vi "FRU PROGRAMMING TOOLKIT - Copy.vi"() -> ()   [LabVIEW 2016]
doc: "This EEPROM example shows a more generalized way to use the I2C basic API to write data. It allows the user to change the following parameters: page size, write delay, the endianness of the address bytes, and the number of bytes in an address.\n\nThe parameters will have the following effects:\n\nTarget Page Size (bytes): This places an additional constraint on the amount of bytes written. The smaller value will be used, and that number of bytes written.\nWrite Delay Between Pages (ms): This will force a mandatory delay after writing bytes to a device.\nData Address Width: This will allow the user to specify the EEPROM Data Address as either 1 or 2 bytes.\nData Address Endianness: This control will change the ordering of the bytes in the EEPROM Data Address, note that this only has an effect if there are 2 bytes in the address.\n\nSince the I2C SDA and SCL lines are open-drain, they must be pulled up to the required reference voltage of your slave by connecting an appropriate resistor (2k-5k) between SCL and your reference voltage and SDA and your reference voltage. For NI-845x Hardware that contain internal pull-ups, you can use these. Otherwise, you need to use external pullups.\n\nFor connection information see the NI-845x Hardware and Software manual and the manual for your specific EEPROM."
uses:
  Type Definitions/I2C Slave Configuration.ctl
  Type Definitions/I2C Device Configuration.ctl
  <vilib>/ni845x/ni845x.llb/ni845xControl.ctl
  Type Definitions/FRU Type.ctl
  Type Definitions/FRU Information.ctl
  Type Definitions/Unique FRU Input.ctl
  Type Definitions/I2C Data Cluster.ctl
  <vilib>/Utility/miscctls.llb/LVRectTypeDef.ctl
  <vilib>/ni845x/ni845x.llb/ni845xI2cConfiguration.ctl
  Type Definitions/I2C Data Address Cluster.ctl
  <vilib>/ni845x/ni845x.llb/NI-845x Close Device Reference.vi
panel:
  out "Front Panel Window:Panel Bounds":T1
  in  "Test Type":enum32{"Standard", "Advanced"}(tab)
  in  "FRU Type":T2
  in  "Unique FRU Input":T3
  in  "I2C Data Cluster":T4={"Address Byte"=0, "Number of Bytes"=0, "Page Size in Bytes"=128, "Data Byte"=[], "Write Delay Between Pages (ms)"=4} {"Data Byte" format="%02x"; "Address Byte" format="%04x"}
  out "PASS":bool
  out "FRU Out":T5
  out "Read Byte":u8[](array[numeric]) format="%02x"
  in  "READ":bool
  in  "Device in":T6="USB0::0x3923::0x7166::01EEC019::RAW"
  out "error out":errorcluster
  in  "INIT":bool
  out "TESTING":bool
  in  "error in (no error)":errorcluster
  in  "EXIT":bool
  in  "CONNECT":bool
  in  "START TEST":bool
  in  "DISCONNECT":bool
  out "Written Byte":u8[](array[numeric]) format="%02x"
  out "Device Out":T6
  in  "I2C Device Configuration":T7={"I²C Pullup Enable"=FALSE, "Timeout Value (ms)"=50000}
  in  "WRITE":bool
  in  "I2C Slave Configuration":T8={"Address"=80, "Clock Rate (kHz)"=100, "Address Size"=0} {"Address Size" items=["7 Bits", "10 Bits"]; "Address" format="%.0x"}
  # "FRU Programming Toolkit"
  # "SOLAHD SCM"
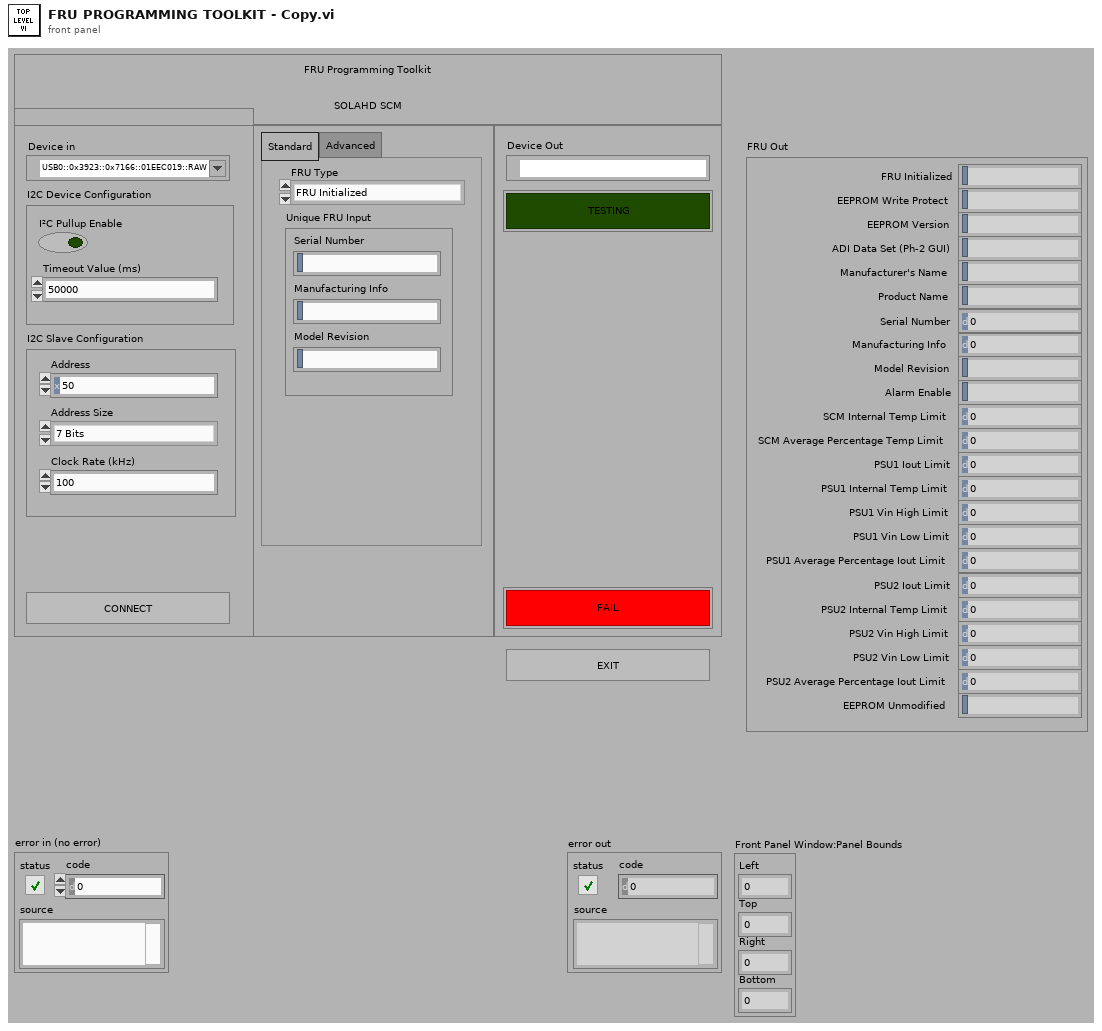
[diagram p1: front panel]
types:
  T1 = typedef "LVRectTypeDef.ctl" = cluster{"Left":i16, "Top":i16, "Right":i16, "Bottom":i16}
  T2 = typedef "FRU Type.ctl" = enum16{"FRU Initialized", "EEROM Write Protect", "EEPROM Version", "ADI Data Set (Ph-2 GUI)", "Manufacturer's Name", "Product Name", "Serial Number", "Manufacturing Info", "Model Revision", "Alarm Enable", "SCM Internal Temp Limit", "SCM Average Percentage Temp Limit", "PSU1 Iout Limit", "PSU1 Internal Temp Limit", "PSU1 Vin High Limit", "PSU1 Vin Low Limit", "PSU1 Average Percentage Iout Limit", "PSU2 Iout Limit", "PSU2 Internal Temp Limit", "PSU2 Vin High Limit", "PSU2 Vin Low Limit", "PSU2 Average Percentage Iout Limit", "EEPROM Unmodified"}
  T3 = typedef "Unique FRU Input.ctl" = cluster{"Serial Number":string, "Manufacturing Info":string, "Model Revision":string}
  T4 = typedef "I2C Data Cluster.ctl" = cluster{"Address Byte":u16, "Number of Bytes":u32, "Page Size in Bytes":u32, "Data Byte":u8[], "Write Delay Between Pages (ms)":u32}
  T5 = typedef "FRU Information.ctl" = cluster{"FRU Initialized":string, "EEPROM Write Protect":string, "EEPROM Version":string, "ADI Data Set (Ph-2 GUI)":string, "Manufacturer's Name":string, "Product Name":string, "Serial Number":u32, "Manufacturing Info":u32, "Model Revision":string, "Alarm Enable":string, "SCM Internal Temp Limit":u32, "SCM Average Percentage Temp Limit":u32, "PSU1 Iout Limit":u32, "PSU1 Internal Temp Limit":u32, "PSU1 Vin High Limit":u32, "PSU1 Vin Low Limit":u32, "PSU1 Average Percentage Iout Limit":u32, "PSU2 Iout Limit":u32, "PSU2 Internal Temp Limit":u32, "PSU2 Vin High Limit":u32, "PSU2 Vin Low Limit":u32, "PSU2 Average Percentage Iout Limit":u32, "EEPROM Unmodified":string}
  T6 = typedef "ni845xControl.ctl" = refnum<k21>
  T7 = typedef "I2C Device Configuration.ctl" = cluster{"I²C Pullup Enable":bool, "Timeout Value (ms)":u32}
  T8 = typedef "I2C Slave Configuration.ctl" = cluster{"Address":u16, "Clock Rate (kHz)":u16, "Address Size":i32}
  T9 = typedef "ni845xI2cConfiguration.ctl" = refnum<k20>
  T10 = typedef "I2C Data Address Cluster.ctl" = cluster{"Data Address Endianness":bool, " Data Address Width":enum16{"1 Byte", "2 Byte"}}
  T11 = enum16{"Always On", "Always Off", "Off While Running"}
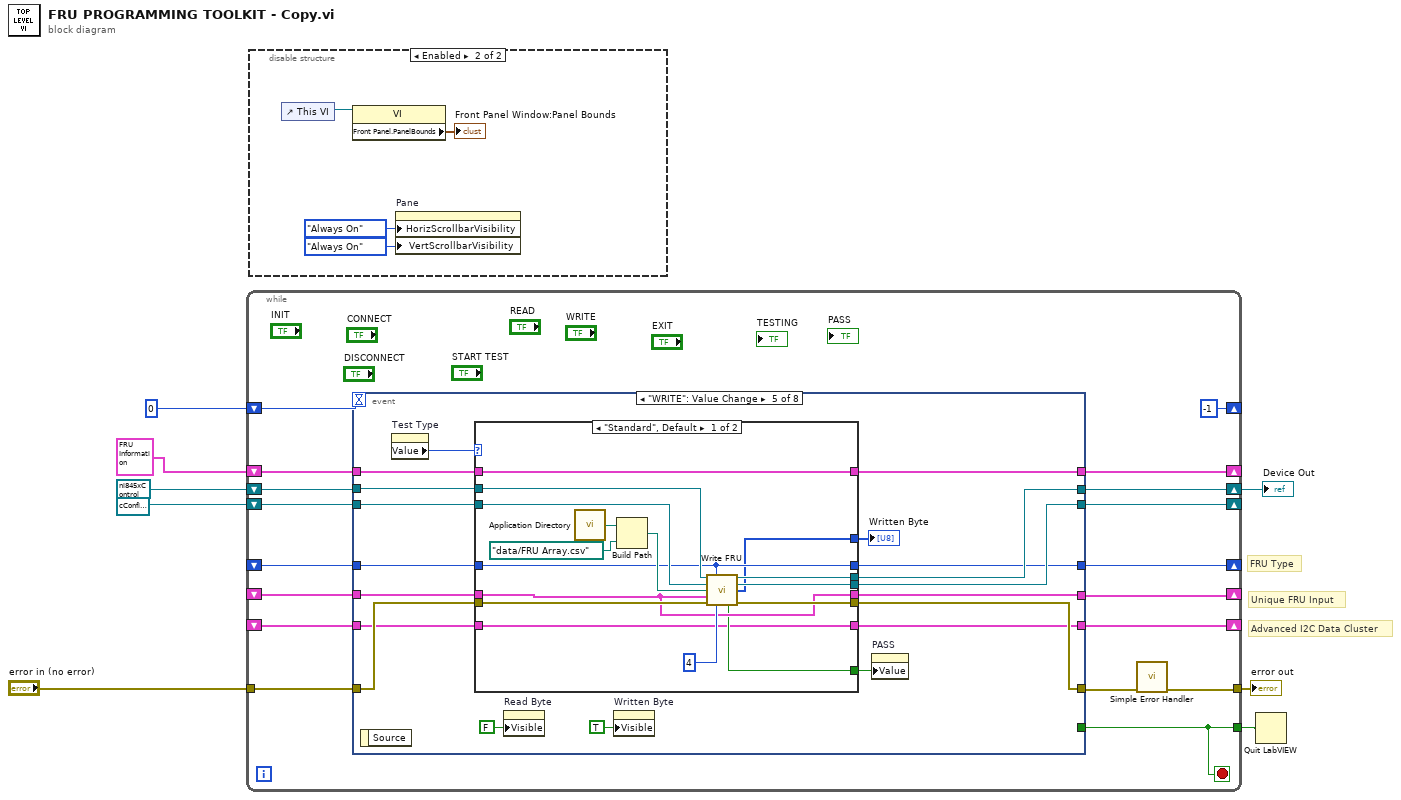
[diagram p0: block diagram]
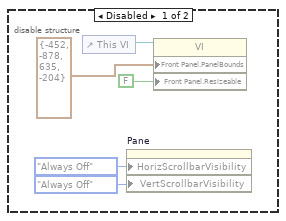
[diagram p2: hidden frame]
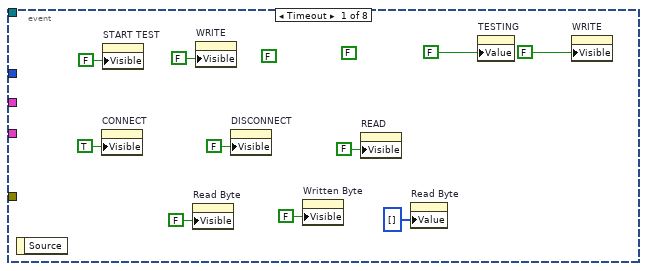
[diagram p3: hidden frame]
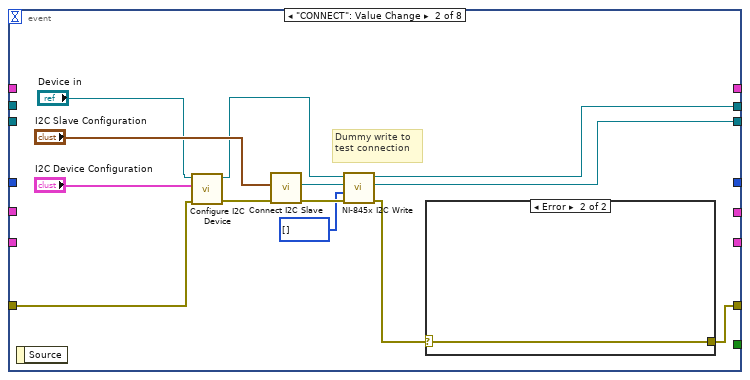
[diagram p4: hidden frame]
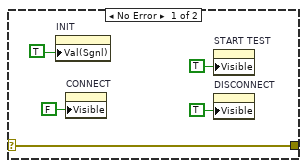
[diagram p5: hidden frame]
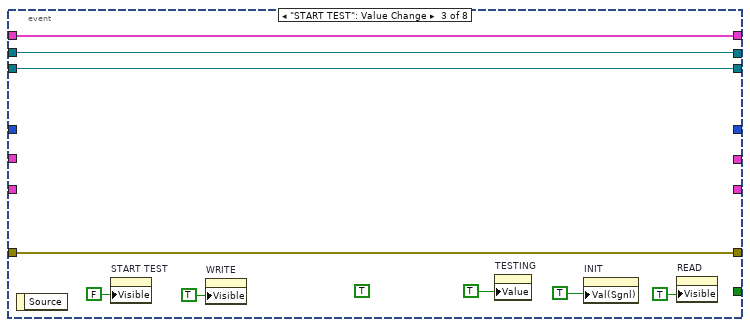
[diagram p6: hidden frame]
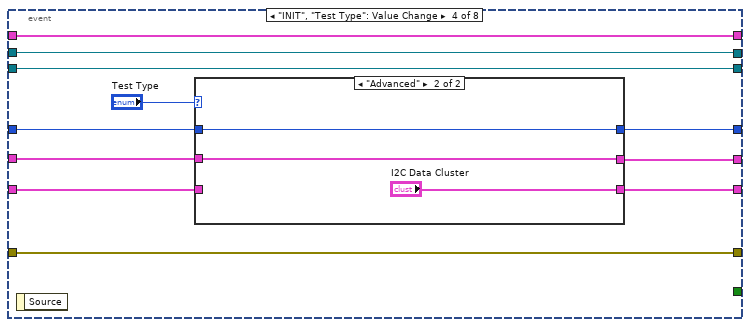
[diagram p7: hidden frame]
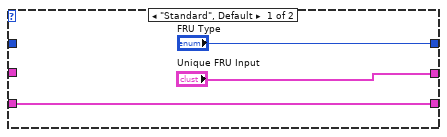
[diagram p8: hidden frame]
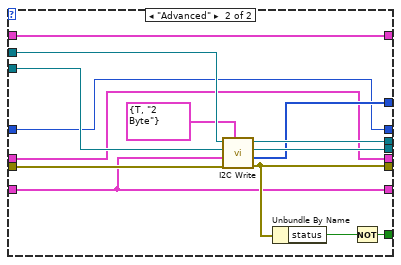
[diagram p9: hidden frame]
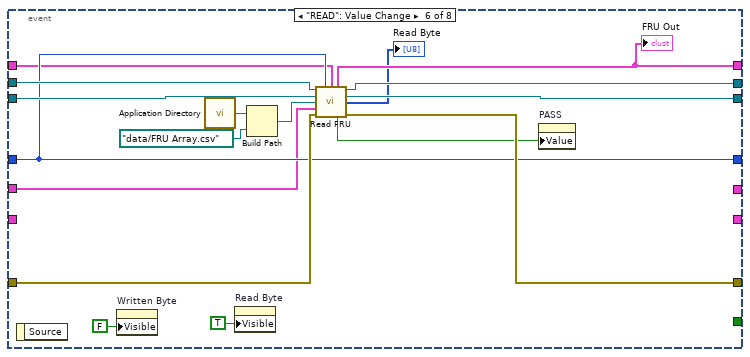
[diagram p10: hidden frame]
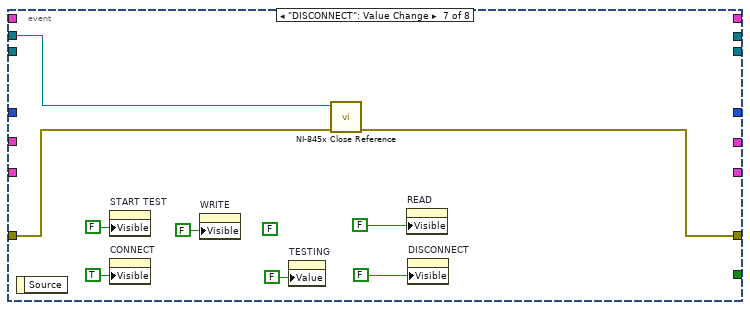
[diagram p11: hidden frame]
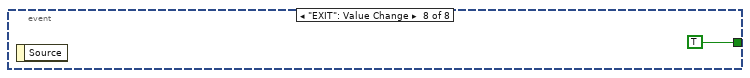
[diagram p12: hidden frame]
diagram:
  # "Advanced I2C Data Cluster"
  # "Unique FRU Input"
  # "FRU Type"
  n1 = while {
    tunnel: [w26] -> w8
    shift-right: [w23] -> _
    shift-left: T9 refnum ("i2c configuration") -> [w20]
    shift-right: [w25] -> w7
    shift-left: T6 refnum ("Device out") -> [w17]
    shift-right: [-1] -> _
    shift-left: 0 -> [w19]
    tunnel: "error in (no error)" -> [w24]
    tunnel: [w21] -> w3
    shift-right: [w16] -> _
    shift-left: T5 {"FRU Initialized"="", "EEPROM Write Protect"="", "EEPROM Version"="", "ADI Data Set (Ph-2 GUI)"="", "Manufacturer's Name"="", "Product Name"="", "Serial Number"=0, "Manufacturing Info"=0, "Model Revision"="", "Alarm Enable"="", "SCM Internal Temp Limit"=0, "SCM Average Percentage Temp Limit"=0, "PSU1 Iout Limit"=0, "PSU1 Internal Temp Limit"=0, "PSU1 Vin High Limit"=0, "PSU1 Vin Low Limit"=0, "PSU1 Average Percentage Iout Limit"=0, "PSU2 Iout Limit"=0, "PSU2 Internal Temp Limit"=0, "PSU2 Vin High Limit"=0, "PSU2 Vin Low Limit"=0, "PSU2 Average Percentage Iout Limit"=0, "EEPROM Unmodified"=""} ("FRU Information Out") -> [w15]
    shift-right: [w14] -> _
    shift-left: _ -> [w13]
    shift-right: [w12] -> _
    shift-left: _ -> [w11]
    shift-right: [w10] -> _
    shift-left: _ -> [w9]
    stop <- w26 stop-if-true
    n2 = event shown="[4] \"WRITE\": Value Change" {
      selector: _ -> [_ _ _ _ _ _ _ _]
      dyn-events: _ -> [_ _ _ _ _ _ _ _]
      timeout: w19 -> [_ _ _ _ _ _ _ _]
      tunnel: [_ _ _ _ _ _ _ TRUE] -> w26
      tunnel: [_ w43 w59 w74 w94 w145 _ _] -> w25
      tunnel: w17 -> [_ _ w59 w74 w96 w147 w149 _]
      tunnel: [_ w39 w64 w75 w97 w141 w152 _] -> w22
      tunnel: w24 -> [_ w46 w64 w75 w100 w144 w148 _]
      tunnel: [_ w42 w56 w71 w93 w137 _ _] -> w23
      tunnel: w20 -> [_ _ w56 w71 w95 w146 _ _]
      tunnel: [_ _ w57 w72 w89 w133 _ _] -> w16
      tunnel: w15 -> [_ _ w57 w72 w90 w135 _ _]
      tunnel: [_ _ _ w73 w88 w136 _ _] -> w14
      tunnel: w13 -> [_ _ _ w66 w92 w136 _ _]
      tunnel: [_ _ _ w70 w86 _ _ _] -> w12
      tunnel: w11 -> [_ _ _ w67 w91 w132 _ _]
      tunnel: [_ _ _ w68 w83 _ _ _] -> w10
      tunnel: w9 -> [_ _ _ w65 w87 _ _ _]
      event Timeout {
        (unwired) FALSE ("Visible")
        (unwired) FALSE ("Visible")
        n3 = event-data() -> ()  [unwired: 1 in, 1 out]
        n4 = property on="CONNECT" class="Bool"("Visible"=TRUE) -> ()  [unwired: 2 in, 2 out]
        n5 = property on="START TEST" class="Bool"("Visible"=FALSE) -> ()  [unwired: 2 in, 2 out]
        n6 = property on="Read Byte" class="Arr (strict)"("Visible"=FALSE) -> ()  [unwired: 2 in, 2 out]
        n7 = property on="WRITE" class="Bool"("Visible"=FALSE) -> ()  [unwired: 2 in, 2 out]
        n8 = property on="DISCONNECT" class="Bool"("Visible"=FALSE) -> ()  [unwired: 2 in, 2 out]
        n9 = property on="Written Byte" class="Arr (strict)"("Visible"=FALSE) -> ()  [unwired: 2 in, 2 out]
        n10 = property on="READ" class="Bool"("Visible"=FALSE) -> ()  [unwired: 2 in, 2 out]
        n11 = property on="Read Byte" class="Arr (strict)"("Value"=u8[] []) -> ()  [unwired: 2 in, 2 out]
        n12 = property on="TESTING" class="Bool (strict)"("Value"=FALSE ("TESTING")) -> ()  [unwired: 2 in, 2 out]
        n13 = property on="WRITE" class="Bool"("Visible"=FALSE) -> ()  [unwired: 2 in, 2 out]
      }
      event "CONNECT": Value Change {
        # "Dummy write to test connection"
        n14 = event-data() -> ()  [unwired: 1 in, 1 out]
        n15 = call "Configure I2C Device.vi"("error in (no error)"=w46, "I2C Device Configuration"="I2C Device Configuration", "Device In"="Device in") -> ("error out"=w47:errorcluster, "Device out"=w41:T6)  [unwired: 7 in]
        n16 = call "Connect I2C Slave.vi"("error in (no error)"=w47, "I2C Slave Configuration"="I2C Slave Configuration") -> ("error out"=w45:errorcluster, "i2c configuration"=w44:T9)  [unwired: 8 in]
        n17 = call <vilib>:"NI-845x I2C Write.vi"("error in (no error)"=w45, "write data"=u8[] [], "i2c configuration in"=w44, "device reference in"=w41) -> ("error out"=w40:errorcluster, "i2c configuration out"=w42:T9, "device reference out"=w43:T6)  [unwired: 5 in]
        n18 = case shown="Error" w40 {
          selector: w40 -> [w54 w55]
          tunnel: [w54 w55] -> w39
          frame No Error {
            n19 = property on="INIT" class="Bool (strict)"("Val(Sgnl)"=TRUE ("Visible")) -> ()  [unwired: 2 in, 2 out]
            n20 = property on="CONNECT" class="Bool"("Visible"=FALSE) -> ()  [unwired: 2 in, 2 out]
            n21 = property on="START TEST" class="Bool"("Visible"=TRUE) -> ()  [unwired: 2 in, 2 out]
            n22 = property on="DISCONNECT" class="Bool"("Visible"=TRUE) -> ()  [unwired: 2 in, 2 out]
          }
          frame Error {
          }
        }
      }
      event "START TEST": Value Change {
        (unwired) TRUE ("Visible")
        n23 = event-data() -> ()  [unwired: 1 in, 1 out]
        n24 = property on="START TEST" class="Bool"("Visible"=FALSE) -> ()  [unwired: 2 in, 2 out]
        n25 = property on="WRITE" class="Bool"("Visible"=TRUE) -> ()  [unwired: 2 in, 2 out]
        n26 = property on="TESTING" class="Bool (strict)"("Value"=TRUE ("TESTING")) -> ()  [unwired: 2 in, 2 out]
        n27 = property on="INIT" class="Bool (strict)"("Val(Sgnl)"=TRUE ("Visible")) -> ()  [unwired: 2 in, 2 out]
        n28 = property on="READ" class="Bool"("Visible"=TRUE) -> ()  [unwired: 2 in, 2 out]
      }
      event "INIT", "Test Type": Value Change {
        n29 = event-data() -> ()  [unwired: 1 in, 1 out]
        n30 = case shown="\"Advanced\"" "Test Type" {
          tunnel: ["FRU Type" w79] -> w73
          tunnel: ["Unique FRU Input" w80] -> w70
          tunnel: [w76 "I2C Data Cluster"] -> w68
          tunnel: w67 -> [_ w80]
          tunnel: w66 -> [_ w79]
          tunnel: w65 -> [w76 _]
          frame "Standard", Default {
          }
          frame "Advanced" {
          }
        }
      }
      event "WRITE": Value Change {
        n31 = event-data() -> ()  [unwired: 1 in, 1 out]
        n32 = property on="Test Type" class="TabCtl (strict)"() -> ("Value"=w82:enum32{"Standard", "Advanced"})  [unwired: 2 in, 2 out]
        n33 = case shown="\"Standard\", Default" w82 {
          tunnel: w100 -> [w116 w122]
          tunnel: [w115 w120] -> w97
          tunnel: w96 -> [w114 w130]
          tunnel: w95 -> [w113 w129]
          tunnel: [w111 w128] -> w94
          tunnel: [w110 w127] -> w93
          tunnel: w92 -> [w105 w119]
          tunnel: w91 -> [w104 w121]
          tunnel: w90 -> [w106 w117]
          tunnel: [w106 w117] -> w89
          tunnel: [w105 w119] -> w88
          tunnel: w87 -> [w101 w118]
          tunnel: [w104 w121] -> w86
          tunnel: [w103 w125] -> w85
          tunnel: [w102 w124] -> w84
          tunnel: [w101 w118] -> w83
          frame "Standard", Default {
            n34 = call <vilib>:"Application Directory.vi"() -> ("Application Directory"=w112:path)
            n35 = Build Path(base path=w112, name or relative path=path "data/FRU Array.csv") -> (appended path=w109:path)
            n36 = call "Write FRU.vi"("device reference in"=w114, "FRU Type"=w105, "i2c configuration in"=w113, "CSV Path"=w109, "Unique FRU Input"=w104, "error in (no error)"=w116, "Write Delay Between Pages (ms)"=u32 4) -> ("device reference out"=w111:T6, "i2c configuration out"=w110:T9, "Data Bytes Written"=w103:u8[], "PASS"=w102:bool, "error out"=w115:errorcluster)  [unwired: 4 in]
          }
          frame "Advanced" {
            n37 = call "I2C Write.vi"("I2C Data Address Cluster"=T10 {"Data Address Endianness"=TRUE, " Data Address Width"=enum."2 Byte"}, "error in (no error)"=w122, "I2C Data Cluster"=w118, "i2c configuration in"=w129, "device reference in"=w130) -> ("error out"=w120:errorcluster, "Data Bytes Written"=w125:u8[], "i2c configuration out"=w127:T9, "device reference out"=w128:T6)  [unwired: 3 in]
            n38 = Unbundle By Name(w120) -> ("status"=w123:bool)
            n39 = Not(x=w123) -> (.not. x?=w124:bool)
          }
        }
        "Written Byte" <- w85
        n40 = property on="Read Byte" class="Arr (strict)"("Visible"=FALSE) -> ()  [unwired: 2 in, 2 out]
        n41 = property on="Written Byte" class="Arr (strict)"("Visible"=TRUE) -> ()  [unwired: 2 in, 2 out]
        n42 = property on="PASS" class="Bool (strict)"("Value"=w84) -> ()  [unwired: 2 in, 2 out]
      }
      event "READ": Value Change {
        n43 = event-data() -> ()  [unwired: 1 in, 1 out]
        n44 = property on="Written Byte" class="Arr (strict)"("Visible"=FALSE) -> ()  [unwired: 2 in, 2 out]
        n45 = call <vilib>:"Application Directory.vi"() -> ("Application Directory"=w140:path)
        n46 = property on="Read Byte" class="Arr (strict)"("Visible"=TRUE) -> ()  [unwired: 2 in, 2 out]
        n47 = Build Path(base path=w140, name or relative path=path "data/FRU Array.csv") -> (appended path=w134:path)
        n48 = call "Read FRU.vi"("Device In"=w147, "FRU Type"=w136, "FRU In"=w135, "i2c configuration in"=w146, "CSV Path"=w134, "Unique FRU Data"=w132, "error in (no error)"=w144) -> ("FRU Out"=w133:T5, "Device Out"=w145:T6, "i2c configuration out"=w137:T9, "Read Byte"=→"Read Byte":u8[], "PASS"=w138:bool, "error out"=w141:errorcluster)  [unwired: 3 in]
        "FRU Out" <- w133
        n49 = property on="PASS" class="Bool (strict)"("Value"=w138) -> ()  [unwired: 2 in, 2 out]
      }
      event "DISCONNECT": Value Change {
        (unwired) FALSE ("Visible")
        n50 = event-data() -> ()  [unwired: 1 in, 1 out]
        n51 = property on="START TEST" class="Bool"("Visible"=FALSE) -> ()  [unwired: 2 in, 2 out]
        n52 = property on="CONNECT" class="Bool"("Visible"=TRUE) -> ()  [unwired: 2 in, 2 out]
        n53 = property on="WRITE" class="Bool"("Visible"=FALSE) -> ()  [unwired: 2 in, 2 out]
        n54 = property on="TESTING" class="Bool (strict)"("Value"=FALSE ("TESTING")) -> ()  [unwired: 2 in, 2 out]
        n55 = call-poly <vilib>:"NI-845x Close Reference.vi"("error in (no error)"=w148, "device reference"=w149) -> ("error out"=w152:errorcluster)  [unwired: 9 out]
        n56 = property on="READ" class="Bool"("Visible"=FALSE) -> ()  [unwired: 2 in, 2 out]
        n57 = property on="DISCONNECT" class="Bool"("Visible"=FALSE) -> ()  [unwired: 2 in, 2 out]
      }
      event "EXIT": Value Change {
        n58 = event-data() -> ()  [unwired: 1 in, 1 out]
      }
    }
    n59 = call <vilib>:"Simple Error Handler.vi"("error in (no error)"=w22) -> ("error out"=w21:errorcluster)  [unwired: 4 in, 4 out]
  }
  "Device Out" <- w7
  "error out" <- w3
  n60 = disable-structure shown="Enabled" {
    frame Disabled {
      n61 = control-ref of="This VI"() -> (w162:refnum<vi>)
      n62 = property on="Pane" class="Pane"("HorizScrollbarVisibility"=T11."Always Off" ("Horizontal Scrollbar Visibility"), "VertScrollbarVisibility"=T11."Always Off" ("Horizontal Scrollbar Visibility")) -> ()  [unwired: 2 in, 2 out]
      n63 = property class="VI"(reference=w162, "Front Panel.PanelBounds"=T1 {"Left"=-452, "Top"=-878, "Right"=635, "Bottom"=-204} ("Front Panel Window:Panel Bounds"), "Front Panel.Resizeable"=FALSE ("Front Panel Window:Resizable")) -> ()  [unwired: 1 in, 2 out]
    }
    frame Enabled {
      n64 = control-ref of="This VI"() -> (w163:refnum<vi>)
      n65 = property class="VI"(reference=w163) -> ("Front Panel.PanelBounds"=→"Front Panel Window:Panel Bounds":T1)  [unwired: 1 in, 2 out]
      n66 = property on="Pane" class="Pane"("HorizScrollbarVisibility"=T11."Always On" ("Horizontal Scrollbar Visibility"), "VertScrollbarVisibility"=T11."Always On" ("Horizontal Scrollbar Visibility")) -> ()  [unwired: 2 in, 2 out]
    }
  }
  n67 = Quit LabVIEW(quit? (T)=w8) -> ()
